vi "Send.vi"(1 "entrée d'erreur (pas d'erreur)":errorcluster, 2 "tableau d'octets non signés":u8[](array[numeric]), 3 "Type":u8, 4 "Nom de ressource VISA":refnum<visa-resource-name>) -> (0 "sortie d'erreur":errorcluster)   [LabVIEW 2010]
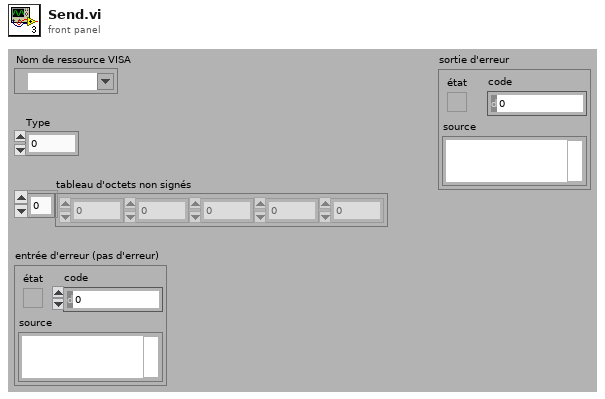
[diagram p1: front panel]
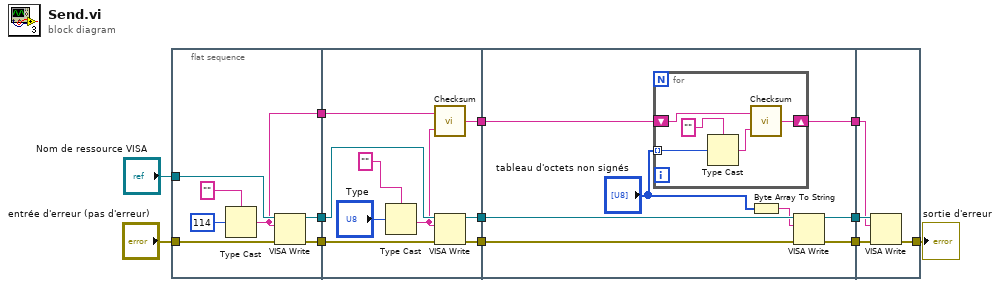
[diagram p0: block diagram]
diagram:
  n1 = flat-sequence {
    tunnel: "Nom de ressource VISA" -> [w19]
    tunnel: "entrée d'erreur (pas d'erreur)" -> [w18]
    tunnel: [w17] -> w12
    tunnel: [w16] -> w11
    tunnel: [w13] -> w10
    tunnel: w12 -> [w28]
    tunnel: w11 -> [w27]
    tunnel: [w24] -> w9
    tunnel: [w23] -> w8
    tunnel: w10 -> [w22]
    tunnel: [w20] -> w7
    tunnel: w9 -> [w36]
    tunnel: w8 -> [w35]
    tunnel: [w34] -> w6
    tunnel: [w33] -> w5
    tunnel: w7 -> [w31]
    tunnel: [w30] -> w4
    tunnel: w6 -> [w45]
    tunnel: w5 -> [w44]
    tunnel: [w43] -> w3
    tunnel: w4 -> [w42]
    frame #0 {
      n2 = Type Cast(type="", x=u8 114) -> (*(type *) &x=w13:string)
      n3 = VISA Write(VISA resource name=w19, write buffer=w13, error in (no error)=w18) -> (VISA resource name out=w17:refnum<visa-resource-name>, error out=w16:errorcluster)  [unwired: 1 out]
    }
    frame #1 {
      n4 = Type Cast(type="", x="Type") -> (*(type *) &x=w21:string)
      n5 = call "Checksum.vi"("Byte2"=w21, "Byte1"=w22) -> ("chaîne"=w20:string)
      n6 = VISA Write(VISA resource name=w28, write buffer=w21, error in (no error)=w27) -> (VISA resource name out=w23:refnum<visa-resource-name>, error out=w24:errorcluster)  [unwired: 1 out]
    }
    frame #2 {
      n7 = for {
        tunnel: "tableau d'octets non signés" -> [w39] mode=indexing
        shift-right: [w40] -> w30
        shift-left: w31 -> [w41]
        n8 = Type Cast(type="", x=w39) -> (*(type *) &x=w37:string)
        n9 = call "Checksum.vi"("Byte2"=w37, "Byte1"=w41) -> ("chaîne"=w40:string)
      }
      n10 = Byte Array To String(unsigned byte array="tableau d'octets non signés") -> (string=w29:string)
      n11 = VISA Write(VISA resource name=w35, write buffer=w29, error in (no error)=w36) -> (VISA resource name out=w34:refnum<visa-resource-name>, error out=w33:errorcluster)  [unwired: 1 out]
    }
    frame #3 {
      n12 = VISA Write(VISA resource name=w45, write buffer=w42, error in (no error)=w44) -> (error out=w43:errorcluster)  [unwired: 2 out]
    }
  }
  "sortie d'erreur" <- w3
